vi "Create Build Specification.vi"(8 "error in":errorcluster, 10 "measurement service name":string, 11 "project ref":refnum<vi>) -> (0 "error out":errorcluster, 3 "project ref out":refnum<vi>)   [LabVIEW 2021, in "MeasurementService Editor.lvlib"]
uses:
  MeasurementService Editor.lvlib
  <vilib>/AppBuilder/AB_API/common/AB_API Primary Exclusions.ctl
  <vilib>/AppBuilder/AB_Source_Property_WindowRunTimePosition.ctl
  NI_AB_API_EXE_Extensions/NI_AB_API_EXE_Extensions.lvclass
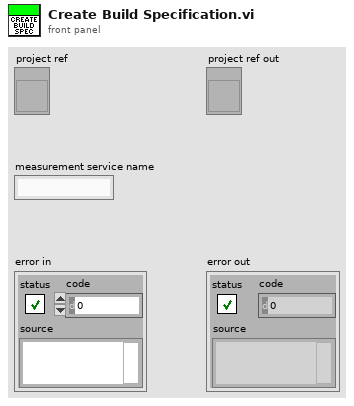
[diagram p1: front panel]
types:
  T1 = typedef "AB_Source_Property_WindowRunTimePosition.ctl" = enum16{"Unchanged", "Centered", "Maximized", "Minimized"}
  T2 = typedef "AB_API Primary Exclusions.ctl" = cluster{"Disconnect type definitions":bool, "Remove unused polymorphic VI instances":bool, "Remove unused members of project libraries":bool, "Modify project library file after removing unused members":bool}
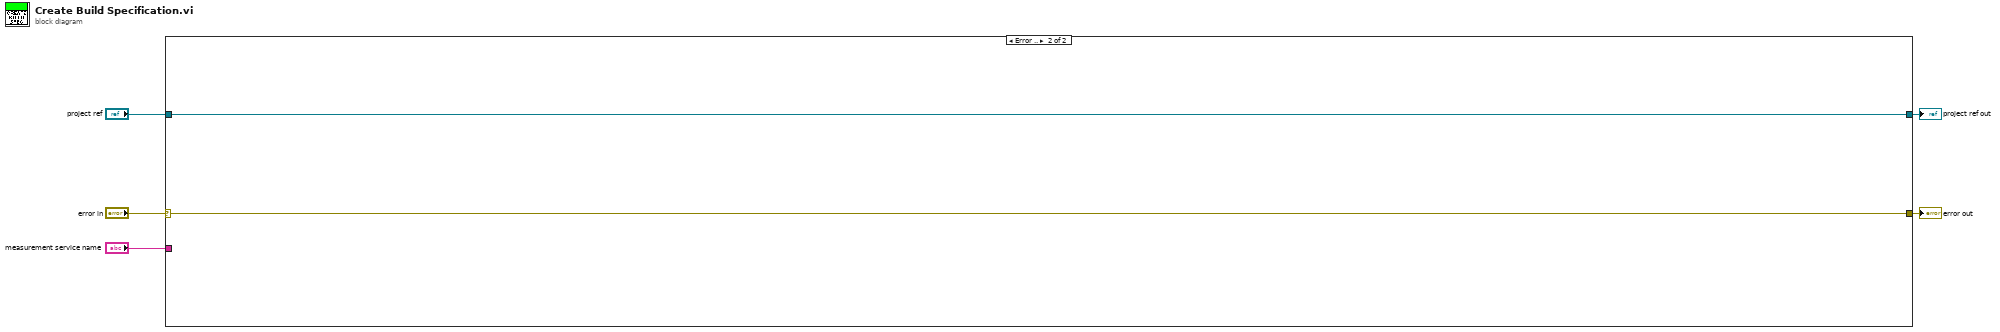
[diagram p0: block diagram]
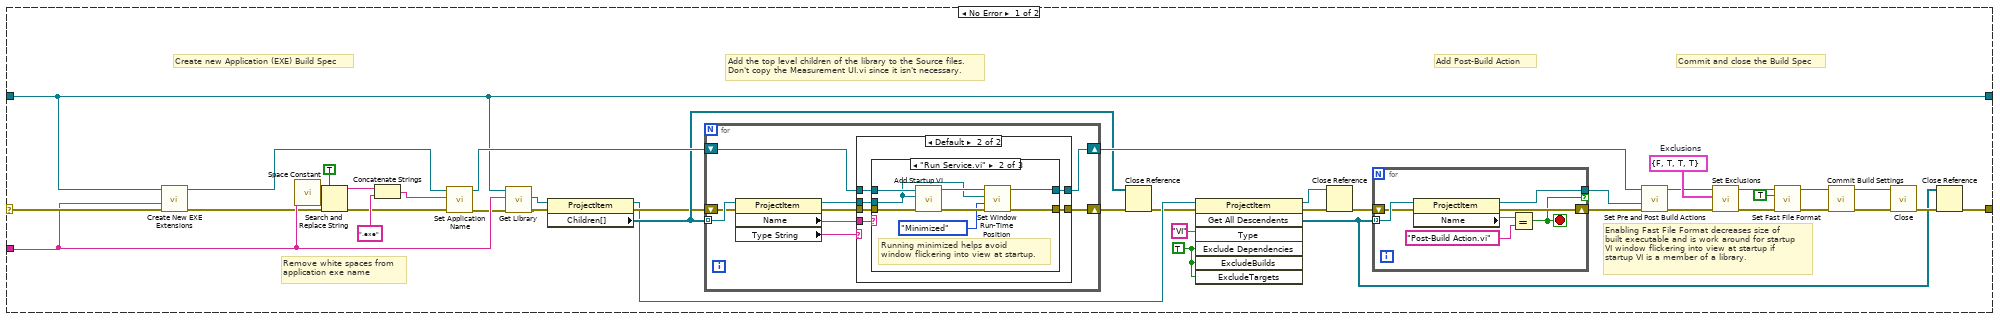
[diagram p2: hidden frame]
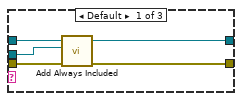
[diagram p4: hidden frame]
diagram:
  n1 = case shown="Error .." "error in" {
    selector: "error in" -> [w46 w87]
    tunnel: "project ref" -> [w6 w86]
    tunnel: "measurement service name" -> [w27 _]
    tunnel: [w18 w87] -> w4
    tunnel: [w6 w86] -> w1
    frame No Error {
      w30 = T2 {"Disconnect type definitions"=FALSE, "Remove unused polymorphic VI instances"=TRUE, "Remove unused members of project libraries"=TRUE, "Modify project library file after removing unused members"=TRUE}  # Exclusions
      w33 = TRUE ("ExcludeDependencies")
      # "Enabling Fast File Format decreases size of\nbuilt executable and is work around for startup\nVI window flickering into view at startup if\nstartup VI is a member of a library."
      # "Remove white spaces from application exe name"
      # "Create new Application (EXE) Build Spec"
      # "Commit and close the Build Spec"
      # "Add Post-Build Action"
      # "Add the top level children of the library to the Source files.\nDon't copy the Measurement UI.vi since it isn't necessary."
      n2 = call "Create New EXE Extensions.vi"("error in (no error)"=w46, "Build specification name"=w27, "Project Refnum"=w6) -> ("error out"=w12:errorcluster, "NI_AB_API_Build out"=w13:refnum<class "NI_AB_API_EXE_Extensions.lvclass">)  [unwired: 7 in]
      n3 = call <vilib>:"Space Constant.vi"() -> ("String"=w44:string)
      n4 = Search and Replace String(replace all?=TRUE ("replace all? (F)"), input string=w27, search string=w44, error in=w12) -> (result string=w43:string, error out=w38:errorcluster)  [unwired: 4 in, 2 out]
      n5 = Concatenate Strings(w43, ".exe" ("string")) -> (w41:string)
      n6 = call-dynamic "Set Application Name.vi"("error in (no error)"=w38, "Application file name"=w41, "EXE in"=w13) -> ("error out"=w24:errorcluster, "EXE out"=w40:refnum<class "NI_AB_API_EXE_Extensions.lvclass">)  [unwired: 7 in]
      n7 = call "Get Library.vi"("error in (no error)"=w24, "library name"=w27, "project ref"=w6) -> ("error out"=w26:errorcluster, "library item"=w25:refnum<vi>)  [unwired: 5 in, 2 out]
      n8 = property class="ProjectItem"(reference=w25, error in=w26) -> (reference out=w15:refnum<vi>, error out=w16:errorcluster, "Children[]"=w23:refnum<vi>[])
      n9 = for {
        tunnel: w23 -> [w62] mode=indexing
        shift-right: [w58] -> w39
        shift-left: w40 -> [w60]
        shift-right: [w55] -> w35
        shift-left: w16 -> [w57]
        n10 = property class="ProjectItem"(reference=w62, error in=w57) -> (reference out=w59:refnum<vi>, error out=w56:errorcluster, "Name"=w61:string, "Type String"=w54:string)
        n11 = case shown="Default" w54 {
          tunnel: w61 -> [_ w70]
          tunnel: w60 -> [w64 w69]
          tunnel: w59 -> [_ w68]
          tunnel: [w64 w67] -> w58
          tunnel: w56 -> [w63 w66]
          tunnel: [w63 w65] -> w55
          frame "Folder" {
          }
          frame Default {
            n12 = case shown="\"Run Service.vi\"" w70 {
              tunnel: w69 -> [w75 w83 w85]
              tunnel: w68 -> [w74 w77 _]
              tunnel: [w73 w80 w85] -> w67
              tunnel: w66 -> [w72 w82 w84]
              tunnel: [w71 w78 w84] -> w65
              frame Default {
                n13 = call-dynamic "Add Always Included.vi"("error in (no error)"=w72, "ProjectItem Refnum"=w74, "EXE in"=w75) -> ("error out"=w71:errorcluster, "EXE out"=w73:refnum<class "NI_AB_API_EXE_Extensions.lvclass">)  [unwired: 7 in]
              }
              frame "Run Service.vi" {
                # "Running minimized helps avoid\nwindow flickering into view at startup."
                n14 = call-dynamic "Add Startup VI.vi"("error in (no error)"=w82, "ProjectItem Refnum"=w77, "EXE in"=w83) -> ("error out"=w79:errorcluster, "EXE out"=w81:refnum<class "NI_AB_API_EXE_Extensions.lvclass">)  [unwired: 7 in]
                n15 = call "Set Window Run-Time Position.vi"("error in (no error)"=w79, "Window Run-Time Position"=AB_Source_Property_WindowRunTimePosition."Minimized", "ProjectItem Refnum"=w77, "NI_AB_API_EXE_Extensions in"=w81) -> ("error out"=w78:errorcluster, "NI_AB_API_EXE_Extensions out"=w80:refnum<class "NI_AB_API_EXE_Extensions.lvclass">)  [unwired: 6 in]
              }
              frame "Measurement UI.vi" {
              }
            }
          }
        }
      }
      n16 = Close Reference(reference=w23, error in (no error)=w35) -> (error out=w14:errorcluster)
      n17 = invoke class="ProjectItem" method="Get All Descendents"(reference=w15, error in=w14, "Type"="VI", "Exclude Dependencies"=w33, "ExcludeBuilds"=w33, "ExcludeTargets"=w33) -> (reference out=w22:refnum<vi>, error out=w21:errorcluster, "All Descendents"=w17:refnum<vi>[])  [unwired: 1 in, 4 out]
      n18 = Close Reference(reference=w22, error in (no error)=w21) -> (error out=w20:errorcluster)
      n19 = for {
        tunnel: w17 -> [w53] mode=indexing
        shift-right: [w50] -> w31
        shift-left: w20 -> [w48]
        tunnel: [w49] -> w32 if=w47
        stop <- w47 stop-if-true
        n20 = property class="ProjectItem"(reference=w53, error in=w48) -> (reference out=w49:refnum<vi>, error out=w50:errorcluster, "Name"=w51:string)
        n21 = Equal?(x=w51, y="Post-Build Action.vi") -> (x = y?=w47:bool)
      }
      n22 = call-dynamic "Set Pre and Post Build Actions.vi"("error in (no error)"=w31, "Post Build Action VI"=w32, "Build in"=w39) -> ("error out"=w28:errorcluster, "Build out"=w29:refnum<class "NI_AB_API_EXE_Extensions.lvclass">)  [unwired: 7 in]
      n23 = call-dynamic "Set Exclusions.vi"("error in (no error)"=w28, "Exclusions"=w30, "EXE in"=w29) -> ("error out"=w9:errorcluster, "EXE out"=w11:refnum<class "NI_AB_API_EXE_Extensions.lvclass">)  [unwired: 7 in]
      n24 = call "Set Fast File Format.vi"("error in (no error)"=w9, "Enable Fast File Format"=TRUE, "NI_AB_API_EXE_Extensions in"=w11) -> ("error out"=w8:errorcluster, "NI_AB_API_EXE_Extensions out"=w10:refnum<class "NI_AB_API_EXE_Extensions.lvclass">)  [unwired: 7 in]
      n25 = call-dynamic "Commit Build Settings.vi"("error in (no error)"=w8, "EXE in"=w10) -> ("error out"=w36:errorcluster, "EXE out"=w37:refnum<class "NI_AB_API_EXE_Extensions.lvclass">)  [unwired: 8 in]
      n26 = call-dynamic "Close.vi"("error in (no error)"=w36, "EXE in"=w37) -> ("error out"=w19:errorcluster)  [unwired: 9 in]
      n27 = Close Reference(reference=w17, error in (no error)=w19) -> (error out=w18:errorcluster)
    }
    frame Error {
    }
  }
  "error out" <- w4
  "project ref out" <- w1
